vi "GetChanOnAndConfigStatus.vi"(8 "error in":errorcluster, 11 "VISA resource name":refnum<visa-resource-name>) -> (0 "error out":errorcluster, 1 "Channel on and configured status binary":string, 2 "Channel on and configured status string":string, 3 "VISA resource name out":refnum<visa-resource-name>)   [LabVIEW 2023, in "Thermotron 8800.lvlib"]
doc: "CHST\nCommand name: Channel on and configured status\nCommand type: System status\nDescription: The 8800 sends a two-byte coded integer describing the channel on and\nconfiguration status.\nByte 1 = channel on status: Bits 0 through 7 indicate the on status of channels 1\nthrough 8 respectively. The 8800 sets the bit for each channel that is on.\nByte 2 = channel configured status: Bits 8 through 15 indicate the configured status\nof channels 1 through 8 respectively. The 8800 sets the bit for each channel that is\nconfigured.\nSyntax: CHST?\nData type: Coded integer\nQuery example: CHST?\n8800 response: 769 (Binary value 00000011 00000001. This indicates that channels 1 and 2 are\nconfigured and that channel 1 is on.)"
uses:
  Thermotron 8800.lvlib
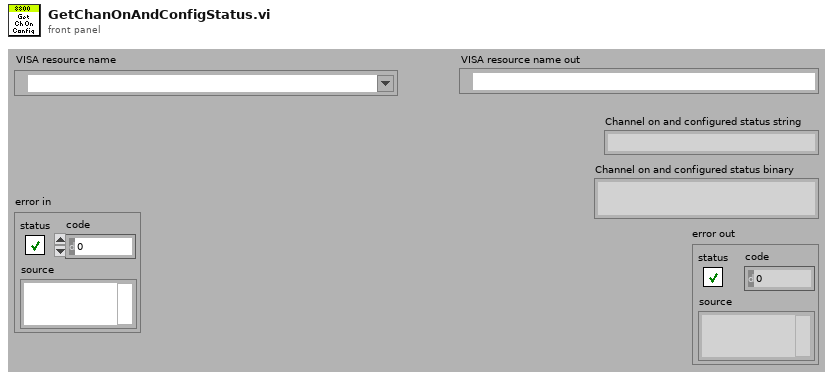
[diagram p1: front panel]
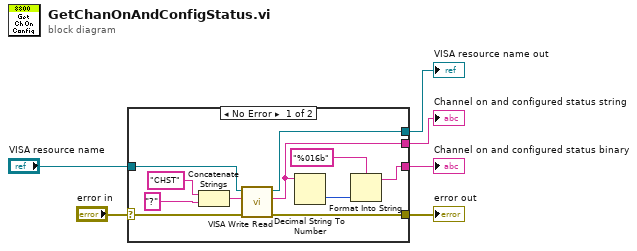
[diagram p0: block diagram]
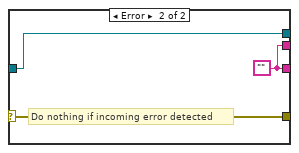
[diagram p2: hidden frame]
diagram:
  n1 = case shown="No Error" "error in" {
    selector: "error in" -> [w11 w19]
    tunnel: "VISA resource name" -> [w12 w20]
    tunnel: [w10 w19] -> w4
    tunnel: [w9 w20] -> w3
    tunnel: [w8 w18] -> w2
    tunnel: [w7 w18] -> w1
    frame No Error {
      n2 = Concatenate Strings("CHST" ("8800 Command"), "?" ("8800 Command")) -> (w13:string)
      n3 = call "VISA Write Read.vi"("error in (no error)"=w11, "8800 Command"=w13, "VISA Refnum in"=w12) -> ("error out"=w10:errorcluster, "read buffer"=w8:string, "VISA Refnum out"=w9:refnum<visa-resource-name>)  [unwired: 6 in]
      n4 = Decimal String To Number(string=w8) -> (number=w16:i32)  [unwired: 2 in, 1 out]
      n5 = Format Into String(format string="%016b", w16) -> (resulting string=w7:string)  [unwired: 2 in, 1 out]
    }
    frame Error {
      w18 = ""
      # "Do nothing if incoming error detected"
    }
  }
  "error out" <- w4
  "VISA resource name out" <- w3
  "Channel on and configured status string" <- w2
  "Channel on and configured status binary" <- w1
